vi "MongoDB.DocumentCount.vi"(8 "error in (no error)":errorcluster, 11 "MongoDB.Collection in":refnum<class "MongoDB.Collection.lvclass">) -> (0 "error out":errorcluster, 2 "Count":i64, 3 "MongoDB.Collection out":refnum<class "MongoDB.Collection.lvclass">)   [LabVIEW 2014, in "MongoDB.Collection.lvclass"]
uses:
  MongoDB.Collection.lvclass
  MongoDB.Collection.lvclass/MongoDB.Collection.ctl
  C:/MongoData/Drivers/mongo-csharp-driver-2.0.0-beta4/mongo-csharp-driver-2.0.0-beta4/src/MongoDB.Driver.Legacy/bin/Release/MongoDB.Driver.Legacy.dll
  MongoData/Drivers/mongo-csharp-driver-2.0.0-beta4/mongo-csharp-driver-2.0.0-beta4/src/MongoDB.Driver.Legacy/bin/Release/MongoDB.Driver.Legacy.dll
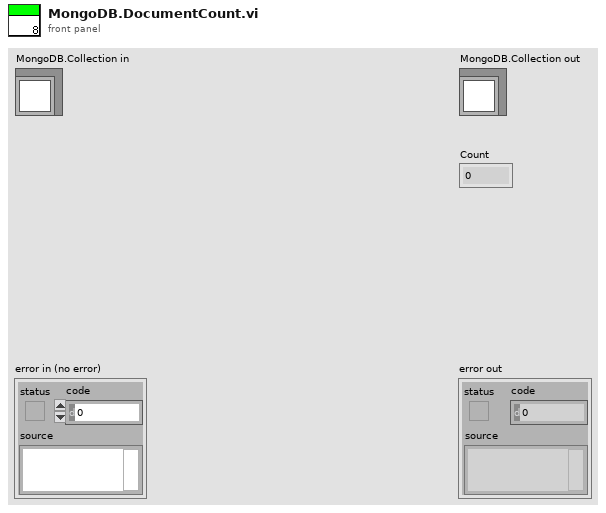
[diagram p1: front panel]
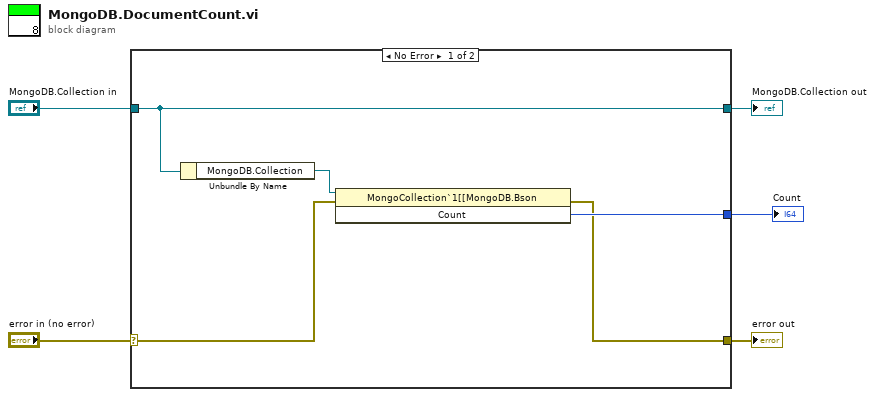
[diagram p0: block diagram]
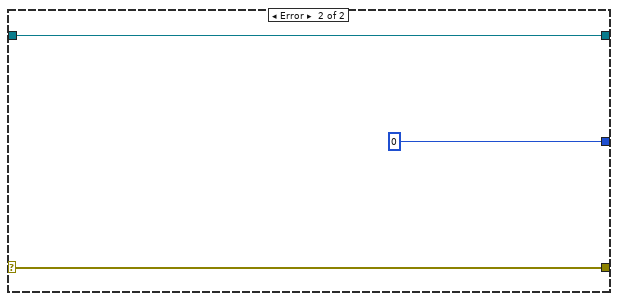
[diagram p2: hidden frame]
diagram:
  n1 = case shown="No Error" "error in (no error)" {
    selector: "error in (no error)" -> [w8 w13]
    tunnel: [w6 w13] -> w4
    tunnel: [w10 w12] -> w2
    tunnel: "MongoDB.Collection in" -> [w10 w12]
    tunnel: [w7 i64 0 ("Count")] -> w1
    frame No Error {
      n2 = Unbundle By Name(w10) -> ("MongoDB.Collection"=w9:refnum<k24>)
      n3 = invoke class="MongoCollection`1[[MongoDB.Bson" method="Count"(reference=w9, error in=w8) -> (error out=w6:errorcluster, "Count"=w7:i64)  [unwired: 1 in, 1 out]
    }
    frame Error {
    }
  }
  "error out" <- w4
  "MongoDB.Collection out" <- w2
  "Count" <- w1
